vi "Read Message Data.lvclass.vi"(8 "error in (no error)":errorcluster, 11 "Message Type in":refnum<class "Message Type.lvclass">) -> (0 "error out":errorcluster, 2 "Message Data.lvclass":refnum<class "Message Data.lvclass">, 3 "Message Type out":refnum<class "Message Type.lvclass">)   [LabVIEW 2023, in "Message Type.lvclass"]
uses:
  Message Type.lvclass
  Message Type.lvclass/Message Type.ctl
  Message Data/Message Data.lvclass
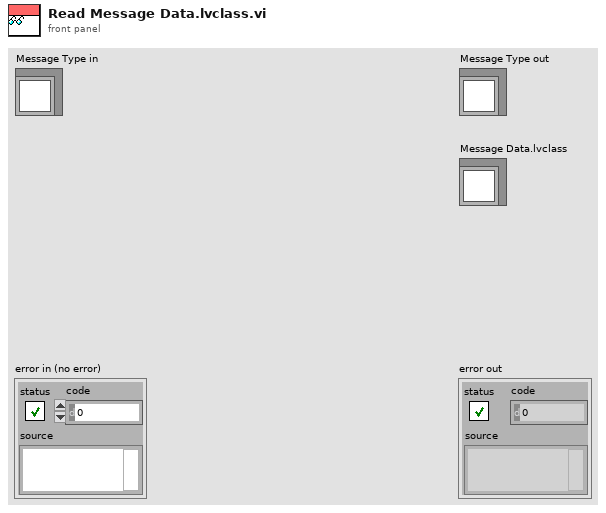
[diagram p1: front panel]
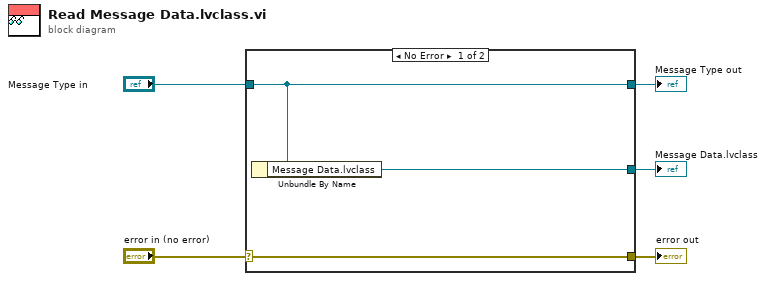
[diagram p0: block diagram]
diagram:
  n1 = case shown="No Error" "error in (no error)" {
    selector: "error in (no error)" -> [w8 w9]
    tunnel: [w8 w9] -> w4
    tunnel: [w7 w10] -> w2
    tunnel: "Message Type in" -> [w7 w10]
    tunnel: [w6 _] -> w1
    frame No Error {
      n2 = Unbundle By Name(w7) -> ("Message Data.lvclass"=w6:refnum<class "Message Data.lvclass">)
    }
    frame Error {
    }
  }
  "error out" <- w4
  "Message Type out" <- w2
  "Message Data.lvclass" <- w1
